vi "F-Anuate.vi"() -> ()   [LabVIEW 2014]
doc: "Use this template to build a VI to use as a subVI."
uses:
  <vilib>/vision/NI_Vision_Development_Module.lvlib
panel:
  out "|F(u,v)H(u,v)|":T1(plugin-control)
  out "g(x,y)":T1(plugin-control)
  out "IF(u,v)I":T1(plugin-control)
  out "f(x,y)":T1(plugin-control)
  # ":: MVi Framework V1.0 ::\nAuthor:Gaoke Yang\nEmail: gaoke.yang@yahoo.com\nWeb: www.mvicontrol.com\nCopyright (C) 2015, MVI Technologies All Rights Reserved"
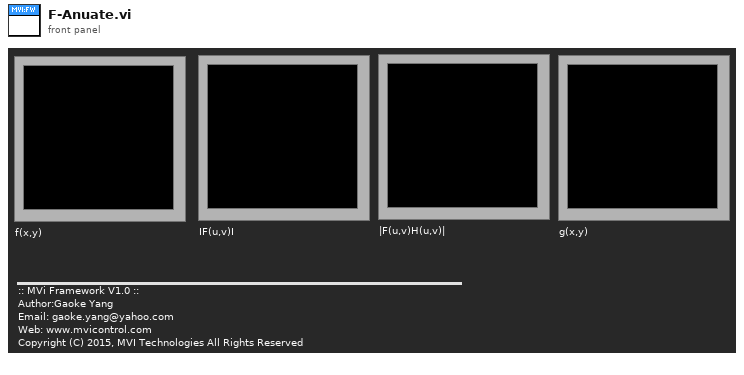
[diagram p1: front panel]
types:
  T1 = typedef "IMAQ Image.ctl" = refnum<image>
  T2 = typedef "Image Type" = u32
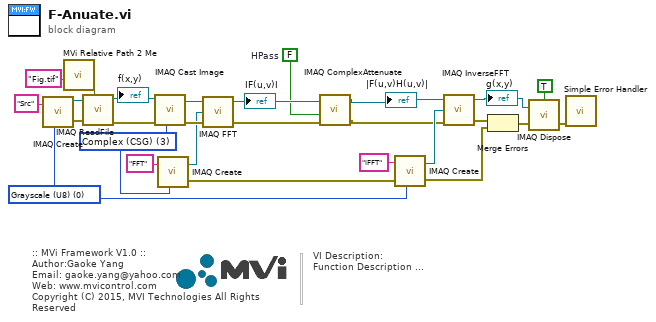
[diagram p0: block diagram]
diagram:
  w1 = FALSE  # HPass
  w6 = T2 0 items=["Grayscale (U8)", "Grayscale (I16)", "Grayscale (SGL)", "Complex (CSG)", "RGB (U32)", "HSL (U32)", "RGB (U64)", "Grayscale (U16)"] ("Image Type")
  w8 = T2 3 items=["Grayscale (U8)", "Grayscale (I16)", "Grayscale (SGL)", "Complex (CSG)", "RGB (U32)", "HSL (U32)", "RGB (U64)", "Grayscale (U16)"] ("Image Type")
  # "VI Description:\nFunction Description ..."
  # ":: MVi Framework V1.0 ::\nAuthor:Gaoke Yang\nEmail: gaoke.yang@yahoo.com\nWeb: www.mvicontrol.com\nCopyright (C) 2015, MVI Technologies All Rights Reserved"
  n1 = call "IMAQ Create"("Image Name"="Src" ("name or relative path"), "Image Type"=w6) -> ("New Image"=w24:T1, "error out"=w23:errorcluster)  [unwired: 2 in, 1 out]
  n2 = call "MVi Relative Path 2 Me.vi"("Relative Path"="Fig.tif" ("name or relative path")) -> ("Appended Dir"=w20:path)  [unwired: 5 in, 1 out]
  n3 = call "IMAQ ReadFile"("File Path"=w20, "error in (no error)"=w23, "Image"=w24) -> ("error out"=w17:errorcluster, "Image Out"=w16:T1)  [unwired: 4 in, 3 out]
  "f(x,y)" <- w16
  n4 = call "IMAQ Cast Image"("Image Type"=w8, "error in (no error)"=w17, "Image Src"=w16) -> ("error out"=w19:errorcluster, "Image Dst Out"=w15:T1)  [unwired: 7 in]
  n5 = call "IMAQ Create"("Image Name"="FFT" ("name or relative path"), "Image Type"=w8) -> ("New Image"=w14:T1, "error out"=w7:errorcluster)  [unwired: 2 in, 1 out]
  n6 = call "IMAQ FFT"("error in (no error)"=w19, "Image Dst"=w14, "Image Src"=w15) -> ("error out"=w2:errorcluster, "Image Dst Out"=w3:T1)  [unwired: 1 in]
  "IF(u,v)I" <- w3
  n7 = call "IMAQ ComplexAttenuate"("error in (no error)"=w2, "Low pass/High pass (Low pass)"=w1, "Image Src"=w3) -> ("error out"=w5:errorcluster, "Image Dst Out"=w4:T1)  [unwired: 2 in]
  "|F(u,v)H(u,v)|" <- w4
  n8 = call "IMAQ Create"("Image Name"="iFFT" ("name or relative path"), "Image Type"=w6, "error in (no error)"=w7) -> ("New Image"=w12:T1, "error out"=w9:errorcluster)  [unwired: 1 in, 1 out]
  n9 = call "IMAQ InverseFFT"("error in (no error)"=w5, "Image Dst"=w12, "Image Src"=w4) -> ("error out"=w11:errorcluster, "Image Dst Out"=w10:T1)  [unwired: 1 in]
  "g(x,y)" <- w10
  n10 = Merge Errors(w11, w9) -> (w18:errorcluster)
  n11 = call "IMAQ Dispose"("All Images? (No)"=TRUE, "Image"=w10, "error in (no error)"=w18) -> ("error out"=w25:errorcluster)  [unwired: 3 out]
  n12 = call <vilib>:"Simple Error Handler.vi"("error in (no error)"=w25) -> ()  [unwired: 1 in, 8 out]
